vi "Init Setting.vi"(8 "error in (no error)":errorcluster, 11 "Controller in":refnum<class "Controller.lvclass">) -> (0 "error out":errorcluster, 3 "Controller out":refnum<class "Controller.lvclass">)   [LabVIEW 2020, in "Controller.lvlib" / "Controller.lvclass"]
uses:
  Controller.lvclass
  <vilib>/ActorFramework/Message/Message.lvclass
  Views/Color Interface/Color/Color Message.lvclass
  MVVM Framework/MVVM Abstruct Controller/MVVM Abstruct Controller/MVVM Abstruct Controller.lvclass/MVVM Abstruct Controller.ctl
  Views/Color Interface/Color/Color Message.lvclass/Color Message.ctl
  <vilib>/ActorFramework/Message Enqueuer/Message Enqueuer.lvclass/Message Enqueuer.ctl
  Views/Color Interface/Color Interface Messages/Set Color Msg/Set Color Msg.lvclass/Set Color Msg.ctl
  Views/Color Interface/Color/Accessors/Write BG Color.vi
  Views/Color Interface/Color/Accessors/Write Fornt Color.vi
  MVVM Framework/MVVM Abstruct Controller/MVVM Abstruct Controller/Accessor/Read ActorMap-Views.vi
  Views/Color Interface/Color Interface Messages/Set Color Msg/Set Color Msg.lvclass
  C:/Program Files (x86)/National Instruments/LabVIEW 2020/vi.lib/ActorFramework/Message/Message.lvclass
  <vilib>/ActorFramework/Message Priority Queue/Priority Enqueue.vi
  Depden On/ActorMap/ActorMap.lvclass
  Controller.lvclass/Controller.ctl
  <vilib>/ActorFramework/Message Enqueuer/Message Enqueuer.lvclass
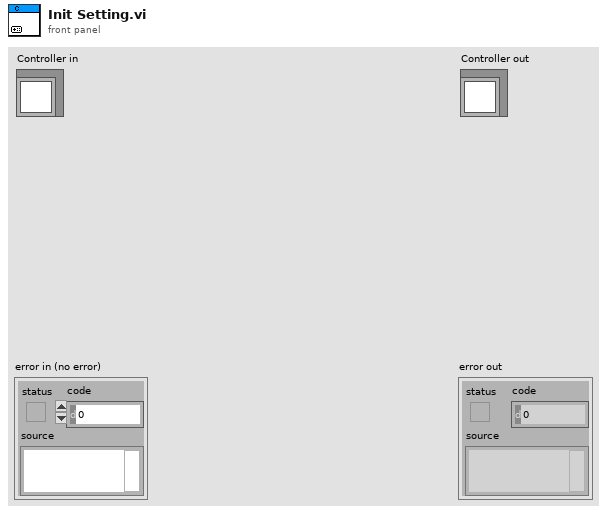
[diagram p1: front panel]
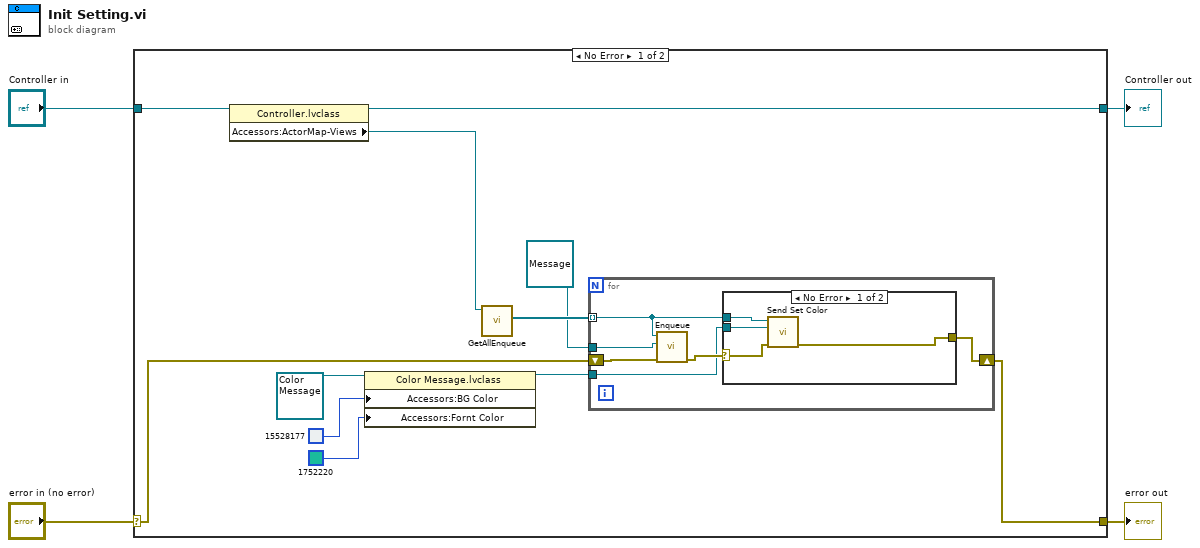
[diagram p0: block diagram]
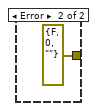
[diagram p2: hidden frame]
diagram:
  n1 = case shown="No Error" "error in (no error)" {
    selector: "error in (no error)" -> [w6 w28]
    tunnel: [w5 w28] -> w3
    tunnel: [w14 w27] -> w1
    tunnel: "Controller in" -> [w15 w27]
    frame No Error {
      n2 = property class="Controller.lvclass"(reference=w15) -> (reference out=w14:refnum<class "Controller.lvclass">, "Accessors:ActorMap-Views"=w11:refnum<class "ActorMap.lvclass">)  [unwired: 1 in, 1 out]
      n3 = property class="Color Message.lvclass"(reference=refnum<class "Color Message.lvclass"> refnum ("Color Message.lvclass"), "Accessors:BG Color"=u32 15528177 ("BG Color"), "Accessors:Fornt Color"=u32 1752220 ("Fornt Color")) -> (reference out=w9:refnum<class "Color Message.lvclass">)  [unwired: 1 in, 1 out]
      n4 = call "GetAllEnqueue.vi"("ActorMap in"=w11) -> ("Enqueues"=w13:refnum<class "Message Enqueuer.lvclass">[])  [unwired: 7 in, 3 out]
      n5 = for {
        tunnel: w13 -> [w20] mode=indexing
        tunnel: refnum<class "Message.lvclass"> refnum ("Message") -> [w19]
        tunnel: w9 -> [w17]
        shift-right: [w21] -> w5
        shift-left: w6 -> [w16]
        n6 = call <vilib>:"Enqueue.vi"("error in (no error)"=w16, "Message"=w19, "Message Enqueuer in"=w20) -> ("error out"=w18:errorcluster)  [unwired: 7 in, 1 out]
        n7 = case shown="No Error" w18 {
          selector: w18 -> [w23 _]
          tunnel: [w25 errorcluster {"status"=FALSE, "code"=0, "source"=""} ("error out")] -> w21
          tunnel: w20 -> [w24 _]
          tunnel: w17 -> [w22 _]
          frame No Error {
            n8 = call "Send Set Color.vi"("error in (no error)"=w23, "Color Message.lvclass"=w22, "Message Enqueuer"=w24) -> ("error out"=w25:errorcluster)  [unwired: 7 in, 1 out]
          }
          frame Error {
          }
        }
      }
    }
    frame Error {
    }
  }
  "error out" <- w3
  "Controller out" <- w1
